vi "AutoNameLancaster.vi"(10 "Custom Folder":string, 11 "User Data Folder":T1) -> (2 "String":string, 3 "created path":path)   [LabVIEW 2014]
uses:
  Users/mbcsslp2/Control 1.ctl
panel:
  in  "Extention":string="dat"
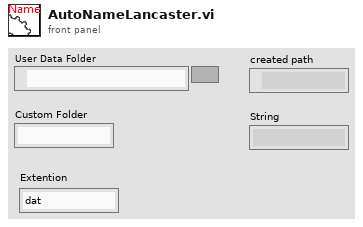
[diagram p1: front panel]
types:
  T1 = typedef "Control 1.ctl" = path
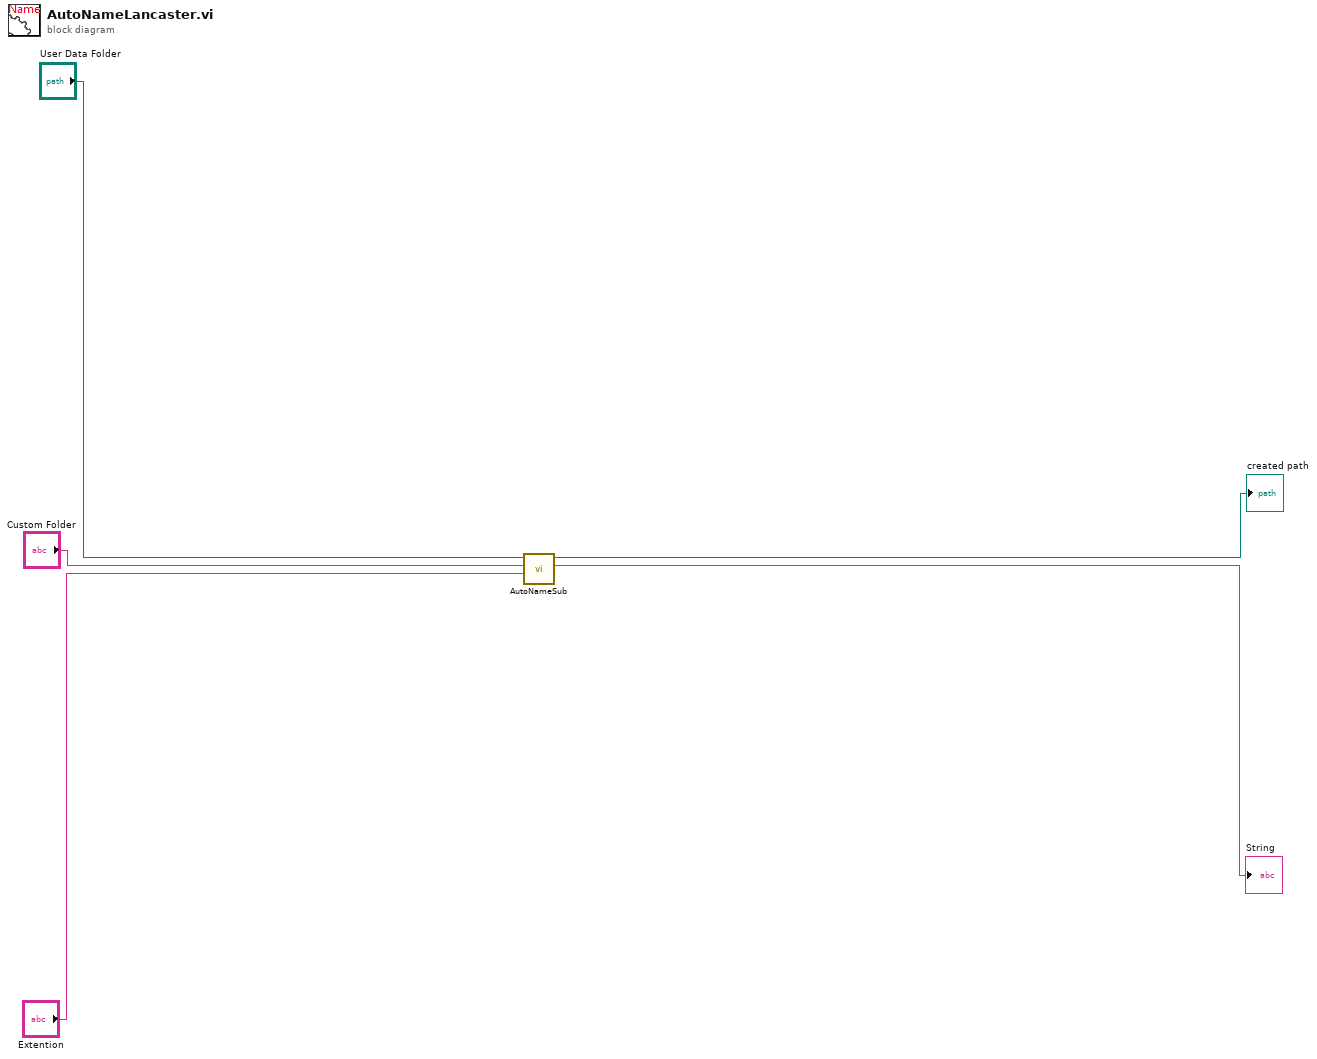
[diagram p0: block diagram]
diagram:
  n1 = call "AutoNameSub.vi"("Extention"="Extention", "Custom Folder"="Custom Folder", "User Data Folder"="User Data Folder") -> ("String"=→"String":string, "created path"=→"created path":path)  [unwired: 7 in]
